vi "force_eqn.vi"(4 "b2_m":dbl, 6 "b1_m":dbl, 8 "error in":errorcluster, 9 "b2_s0":dbl[](array[numeric]), 10 "b1_s0":dbl[](array[numeric])) -> (0 "error out":errorcluster, 2 "r":dbl, 3 "F":dbl[](array[numeric]))   [LabVIEW 2020]
panel:
  out "Fy":dbl
  out "F_mag":dbl
  out "Fx":dbl
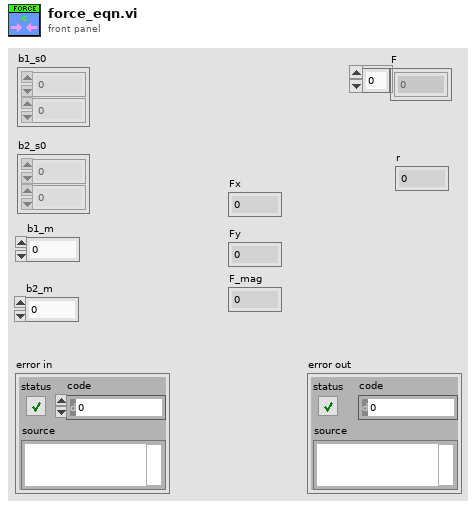
[diagram p1: front panel]
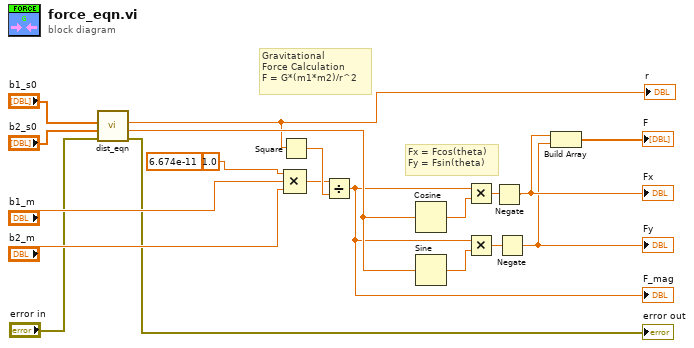
[diagram p0: block diagram]
diagram:
  (unwired) 6.674e-11
  # "Fx = Fcos(theta)\nFy = Fsin(theta)"
  # "Gravitational\nForce Calculation\nF = G*(m1*m2)/r^2"
  n1 = call "dist_eqn.vi"("error in"="error in", "b2_s"="b2_s0", "b1_s"="b1_s0") -> ("error out"=→"error out":errorcluster, "theta"=w8:dbl, "r"=w5:dbl)  [unwired: 6 in]
  "r" <- w5
  n2 = Square(x=w5) -> (x^2=w18:dbl)
  n3 = Compound Arithmetic op=MULTIPLY(1.0, "b1_m", "b2_m") -> (w17:dbl)
  n4 = Divide(x=w17, y=w18) -> (x/y=w7:dbl)
  "F_mag" <- w7
  n5 = Cosine(x=w8) -> (cos(x)=w10:dbl)
  n6 = Sine(x=w8) -> (sin(x)=w9:dbl)
  n7 = Multiply(x=w7, y=w10) -> (x*y=w4:dbl)
  n8 = Multiply(x=w7, y=w9) -> (x*y=w2:dbl)
  n9 = Negate(x=w4) -> (-x=w3:dbl)
  "Fx" <- w3
  n10 = Negate(x=w2) -> (-x=w1:dbl)
  "Fy" <- w1
  n11 = Build Array(w3, w1) -> (→"F":dbl[])
